vi "relative access path.vi"(11 "Oauth2.Salesforce":refnum<class "Oauth2.Salesforce.lvclass">) -> (1 "Token Access Path":string, 2 "Authorization Path":string)   [LabVIEW 2017, in "Oauth2.Salesforce.lvclass"]
uses:
  Oauth2.Salesforce.lvclass
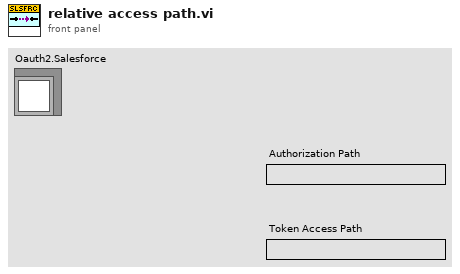
[diagram p1: front panel]
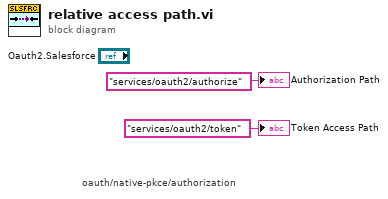
[diagram p0: block diagram]
diagram:
  # "oauth/native-pkce/authorization"
  "Authorization Path" <- "services/oauth2/authorize" ("Authorization Path")
  "Token Access Path" <- "services/oauth2/token" ("Authorization Path")
